vi "test Scaling and Unscaling.vi"(8 "error in (no error)":errorcluster, 11 "TestCase in":refnum<class "BCD.lvclass">) -> (0 "error out":errorcluster, 3 "TestCase out":refnum<class "BCD.lvclass">)   [LabVIEW 2020, in "BCD.lvclass"]
uses:
  BCD.lvclass
  5f41c702-736d-46cb-8ad7-d7a8da9834e5.vi
  e5a9ed8d-a936-4bcd-9e48-8176d125cb75.vi
  5f41c702-736d-46cb-8ad7-d7a8da9834e5.vi/a54b505c-1216-4ef4-8378-3ceda9d188df.vi
  5f41c702-736d-46cb-8ad7-d7a8da9834e5.vi/136dcdcb-2dd3-4a4d-a796-a8f7a3f8e1ac.vi
  e5a9ed8d-a936-4bcd-9e48-8176d125cb75.vi/0a001d06-2809-4638-8d0b-e017d2157007.vi
  BCD Decode Integer.vi
  5f41c702-736d-46cb-8ad7-d7a8da9834e5.vi/a54b505c-1216-4ef4-8378-3ceda9d188df.vi/a7fcce85-1f75-4572-aeaa-ddfd463a7c5f.vi
  BCD Decode Integer.vi/9a65bfc0-0d77-4ef3-ab58-63df1e1caa90.vi
  <vilib>/addons/_JKI Toolkits/VI Tester/TestCase.llb/TestCase.lvclass
  C:/Program Files (x86)/National Instruments/LabVIEW 2020/vi.lib/addons/_JKI Toolkits/VI Tester/TestCase.llb/TestCase.lvclass
panel:
  out "BCD encoded value":bool[](array[boolean])
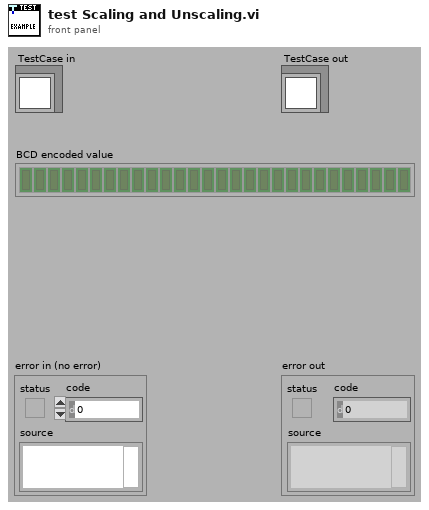
[diagram p1: front panel]
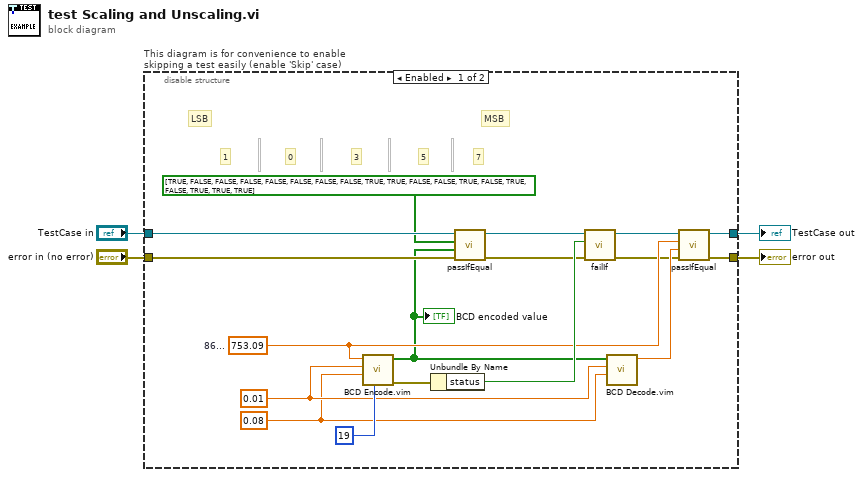
[diagram p0: block diagram]
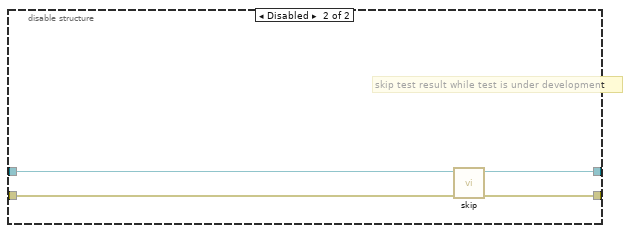
[diagram p2: hidden frame]
diagram:
  n1 = disable-structure "This diagram is for convenience to enable skipping a test easily (enable 'Skip' case)" shown="Enabled" {
    disable-tunnel: "TestCase in" -> [w19 w25]
    disable-tunnel: [w5 w23] -> w1
    disable-tunnel: [w6 w24] -> w3
    disable-tunnel: "error in (no error)" -> [w18 w22]
    frame Enabled {
      w11 = 0.08 ("scale multiplier")
      w12 = 0.01 ("scale multiplier")
      w14 = 753.09  # 86...
      # "MSB"
      # "LSB"
      # "1"
      # "0"
      # "3"
      # "5"
      # "7"
      n2 = call "BCD Encode.vim"("data size (bits)"=19, "scale offset"=w11, "scale multiplier"=w12, "value"=w14) -> ("error out"=w16:errorcluster, "BCD encoded value"=w13:bool[])  [unwired: 5 in, 1 out]
      "BCD encoded value" <- w13
      n3 = Unbundle By Name(w16) -> ("status"=w15:bool)
      n4 = call-dynamic "passIfEqual.vi"("error in (no error)"=w18, "y"=w13, "x"=bool[] [TRUE, FALSE, FALSE, FALSE, FALSE, FALSE, FALSE, FALSE, TRUE, TRUE, FALSE, FALSE, TRUE, FALSE, TRUE, FALSE, TRUE, TRUE, TRUE] ("BCD encoded value"), "TestCase in"=w19) -> ("error out"=w9:errorcluster, "TestCase out"=w10:refnum<class "BCD.lvclass">)  [unwired: 6 in]
      n5 = call-dynamic "failIf.vi"("error in (no error)"=w9, "fail"=w15, "TestCase in"=w10) -> ("error out"=w7:errorcluster, "TestCase out"=w8:refnum<class "BCD.lvclass">)  [unwired: 7 in]
      n6 = call "BCD Decode.vim"("scale offset"=w11, "scale multiplier"=w12, "BCD encoded value"=w13) -> ("value"=w20:dbl)  [unwired: 8 in]
      n7 = call-dynamic "passIfEqual.vi"("error in (no error)"=w7, "y"=w20, "x"=w14, "TestCase in"=w8) -> ("error out"=w6:errorcluster, "TestCase out"=w5:refnum<class "BCD.lvclass">)  [unwired: 6 in]
    }
    frame Disabled {
      # "skip test result while test is under development"
      n8 = call <vilib>:"skip.vi"("error in (no error)"=w22, "TestCase in"=w25) -> ("error out"=w24:errorcluster, "TestCase out"=w23:refnum<class "BCD.lvclass">)  [unwired: 8 in]
    }
  }
  "error out" <- w3
  "TestCase out" <- w1
